vi "test_BuildEvalStr_Boolean.vi"(8 "error in (no error)":errorcluster, 11 "TestCase in":refnum<class "Build Eval Str Test Case.lvclass">) -> (0 "error out":errorcluster, 3 "TestCase out":refnum<class "Build Eval Str Test Case.lvclass">)   [LabVIEW 2018, in "Build Eval Str Test Case.lvclass"]
uses:
  Build Eval Str Test Case.lvclass
  Plugins/Utility/Test Classes/Boolean/Boolean.lvclass
  C:/Users/UKHornP/Documents/Work/Projects/Assert_API/Plugins/Utility/Test Classes/Test.lvclass
  Plugins/Utility/Test Classes/Test Class String IDs.vi
  <vilib>/addons/_JKI Toolkits/VI Tester/TestCase.llb/TestCase.lvclass
  Plugins/Utility/Test Classes/Test.lvclass
  C:/Program Files (x86)/National Instruments/LabVIEW 2018/vi.lib/addons/_JKI Toolkits/VI Tester/TestCase.llb/TestCase.lvclass
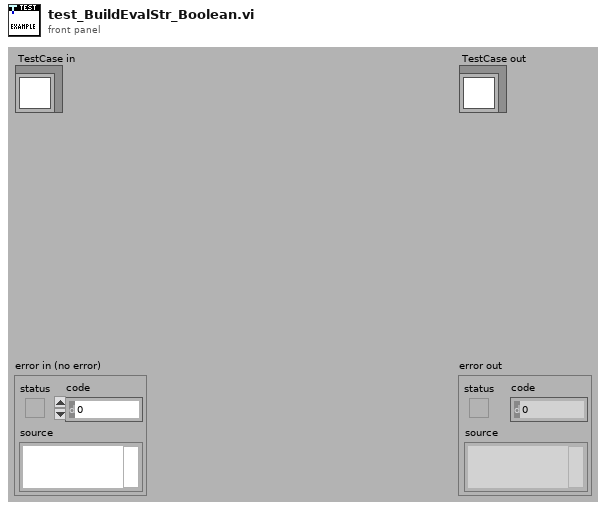
[diagram p1: front panel]
types:
  T1 = cluster{"Comparison Value 1":string, "Comparison Value 2":string, "Invert Result":string, "Assert VI Name":string, "Data Type":string, "Builder User Name":string, "Build Timestamp":string, "Failure Action":string, "Comment":string, "Assert Name":string, "Description":string, "Evaluation String":string, "MD5":string}
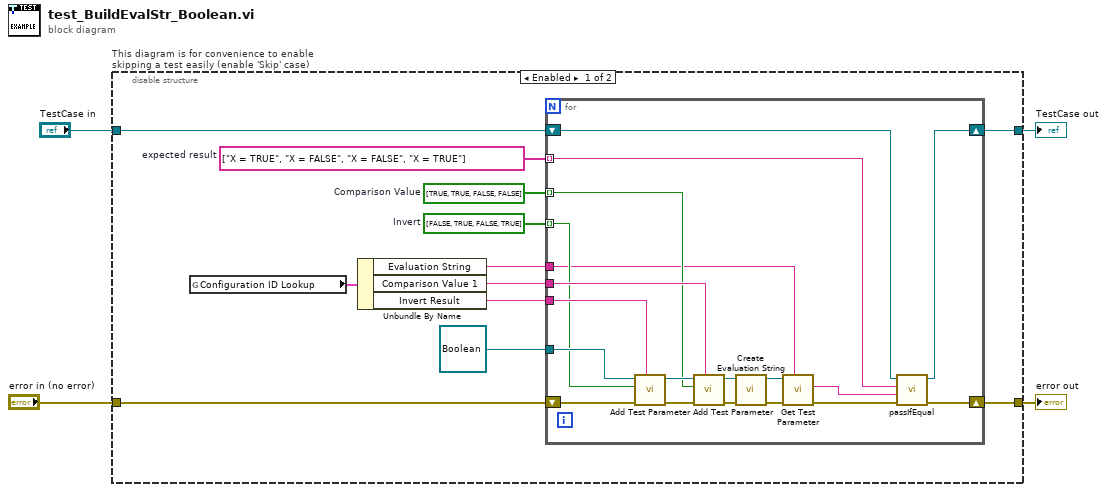
[diagram p0: block diagram]
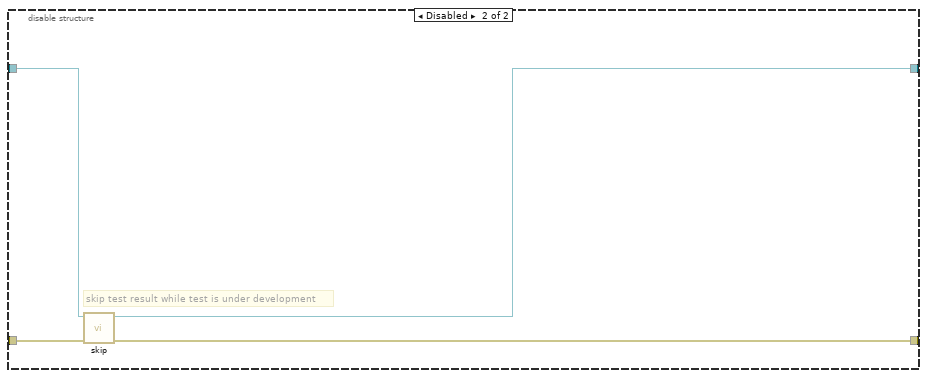
[diagram p2: hidden frame]
diagram:
  n1 = disable-structure "This diagram is for convenience to enable skipping a test easily (enable 'Skip' case)" shown="Enabled" {
    disable-tunnel: "TestCase in" -> [w15 w39]
    disable-tunnel: [w14 w37] -> w1
    disable-tunnel: [w13 w38] -> w3
    disable-tunnel: "error in (no error)" -> [w6 w36]
    frame Enabled {
      w7 = bool[] [TRUE, TRUE, FALSE, FALSE]  # Comparison Value
      w8 = bool[] [FALSE, TRUE, FALSE, TRUE]  # Invert
      w16 = string[] ["X = TRUE", "X = FALSE", "X = FALSE", "X = TRUE"]  # expected result
      n2 = global read "Test Class String IDs.vi" "Configuration ID Lookup"() -> (w11:T1)
      n3 = Unbundle By Name(w11) -> ("Evaluation String"=w5:string, "Comparison Value 1"=w9:string, "Invert Result"=w10:string)
      n4 = for {
        tunnel: w16 -> [w35] mode=indexing
        tunnel: refnum<class "Boolean.lvclass"> refnum ("Boolean.lvclass") -> [w31]
        tunnel: w10 -> [w30]
        tunnel: w9 -> [w29]
        tunnel: w8 -> [w27] mode=indexing
        tunnel: w7 -> [w26] mode=indexing
        tunnel: w5 -> [w18]
        shift-right: [w33] -> w14
        shift-left: w15 -> [w34]
        shift-right: [w32] -> w13
        shift-left: w6 -> [w25]
        n5 = call-dynamic "Add Test Parameter.vi"("Data Value ID"=w30, "error in (no error)"=w25, "Data Value"=w27, "Test in"=w31) -> ("error out"=w24:errorcluster, "Test out"=w28:refnum<class "Boolean.lvclass">)  [unwired: 5 in, 1 out]
        n6 = call-dynamic "Add Test Parameter.vi"("Data Value ID"=w29, "error in (no error)"=w24, "Data Value"=w26, "Test in"=w28) -> ("error out"=w22:errorcluster, "Test out"=w23:refnum<class "Boolean.lvclass">)  [unwired: 5 in, 1 out]
        n7 = call-dynamic "Create Evaluation String.vi"("error in (no error)"=w22, "Boolean in"=w23) -> ("error out"=w21:errorcluster, "Boolean out"=w19:refnum<class "Boolean.lvclass">)  [unwired: 8 in]
        n8 = call "Get Test Parameter.vi"("Data Value ID"=w18, "error in (no error)"=w21, "Test in"=w19) -> ("error out"=w20:errorcluster, "Test Parameter"=w17:string)  [unwired: 6 in, 1 out]
        n9 = call-dynamic "passIfEqual.vi"("error in (no error)"=w20, "y"=w17, "x"=w35, "TestCase in"=w34) -> ("error out"=w32:errorcluster, "TestCase out"=w33:refnum<class "Build Eval Str Test Case.lvclass">)  [unwired: 6 in]
      }
    }
    frame Disabled {
      # "skip test result while test is under development"
      n10 = call <vilib>:"skip.vi"("error in (no error)"=w36, "TestCase in"=w39) -> ("error out"=w38:errorcluster, "TestCase out"=w37:refnum<class "Build Eval Str Test Case.lvclass">)  [unwired: 8 in]
    }
  }
  "error out" <- w3
  "TestCase out" <- w1
